vi "SubVI Tester.vi"() -> ()   [LabVIEW 2015]
uses:
  Control 1.ctl
panel:
  in  "Current Windspeed":dbl
  in  "Max Windspeed":dbl
  out "Weather Data":T1={"Current Temperature"=0.0, "Max Temperature"=0.0, "Min Temperature"=0.0, "Temperature Warning Text"="No Warning", "Temperatur Warning?"=FALSE, "Units"=enum."Fahrenheit", "Current Windspeed"=0.0, "Max Windspeed"=0.0, "Windspeed Warning?"=FALSE, "Windspeed Warning Text"="No Warning"}
  in  "Min Temperature":dbl=10.0
  in  "Max Temperature":dbl=30.0
  in  "Stop":bool
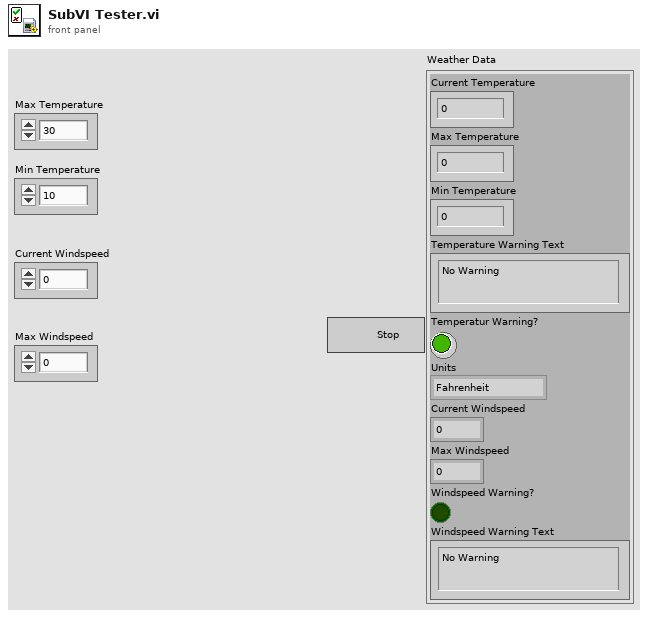
[diagram p1: front panel]
types:
  T1 = typedef "Control 1.ctl" = cluster{"Current Temperature":dbl, "Max Temperature":dbl, "Min Temperature":dbl, "Temperature Warning Text":string, "Temperatur Warning?":bool, "Units":enum16{"Fahrenheit", "Celsius"}, "Current Windspeed":dbl, "Max Windspeed":dbl, "Windspeed Warning?":bool, "Windspeed Warning Text":string}
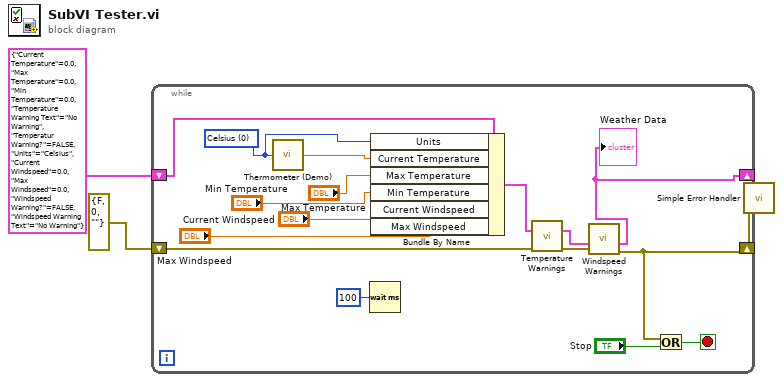
[diagram p0: block diagram]
diagram:
  n1 = while {
    shift-right: [w8] -> w3
    shift-left: errorcluster {"status"=FALSE, "code"=0, "source"=""} ("error out") -> [w12]
    shift-right: [w6] -> _
    shift-left: T1 {"Current Temperature"=0.0, "Max Temperature"=0.0, "Min Temperature"=0.0, "Temperature Warning Text"="No Warning", "Temperatur Warning?"=FALSE, "Units"=enum."Celsius", "Current Windspeed"=0.0, "Max Windspeed"=0.0, "Windspeed Warning?"=FALSE, "Windspeed Warning Text"="No Warning"} ("Weather Data 2") -> [w16]
    stop <- w17 stop-if-true
    w11 = u16 0 items=["Celsius", "Fahrenheit"] ("Units (0: Celsius)")
    n2 = call "Thermometer (Demo).vi"("Units (0: Celsius)"=w11) -> ("Temperature Value"=w15:dbl)
    n3 = Wait (ms)(milliseconds to wait=u32 100) -> ()  [unwired: 1 out]
    n4 = Bundle By Name(cluster=w16, "Units"=w11, "Current Temperature"=w15, "Max Temperature"="Max Temperature", "Min Temperature"="Min Temperature", "Current Windspeed"="Current Windspeed", "Max Windspeed"="Max Windspeed") -> (w10:T1)
    n5 = call "Temperature Warnings.vi"("Weather Data In"=w10, "Error In"=w12) -> ("Weather Data Out"=w7:T1, "Error Out"=w9:errorcluster)  [unwired: 12 in]
    n6 = call "Windspeed Warnings.vi"("Error In"=w9, "Weather Data In"=w7) -> ("Error Out"=w8:errorcluster, "Weather Data Out"=w6:T1)  [unwired: 8 in]
    "Weather Data" <- w6
    n7 = Or(x=w8, y="Stop") -> (x .or. y?=w17:bool)
  }
  n8 = call <vilib>:"Simple Error Handler.vi"("error in (no error)"=w3) -> ()  [unwired: 4 in, 5 out]
